vi "Create DVR.vi"(8 "Error In":errorcluster, 11 "Arithmetic Class":refnum<class "Arithemetic Operation.lvclass">) -> (0 "Error Out":errorcluster, 3 "DVR":refnum<data-value>)   [LabVIEW 2023, in "Arithemetic Operation.lvclass"]
doc: "The method creates a DVR for the given class data."
uses:
  Arithemetic Operation.lvclass
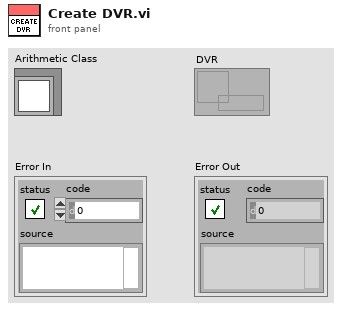
[diagram p1: front panel]
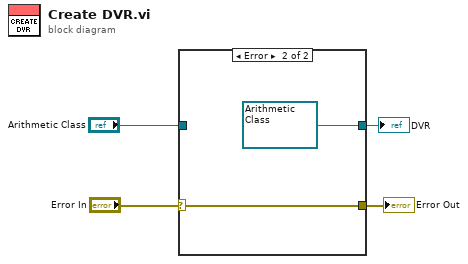
[diagram p0: block diagram]
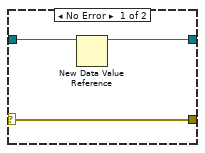
[diagram p2: hidden frame]
diagram:
  n1 = case shown="Error" "Error In" {
    selector: "Error In" -> [w7 w9]
    tunnel: [w7 w9] -> w3
    tunnel: "Arithmetic Class" -> [w6 _]
    tunnel: [w5 refnum<data-value> refnum ("data value reference")] -> w1
    frame No Error {
      n2 = New Data Value Reference(data value=w6) -> (data value reference=w5:refnum<data-value>)  [unwired: 1 in, 1 out]
    }
    frame Error {
    }
  }
  "Error Out" <- w3
  "DVR" <- w1
